vi "command_publisher.vi"() -> ()   [LabVIEW 2016]
uses:
  ts_sallv_exa/DataTypes/command_start.ctl
  ts_sallv_exa/SALLV_EXA.lvlib
panel:
  out "function return":i32
  out "waitComplete":cluster{"cmdSeqNum":i32, "timeout":u32}
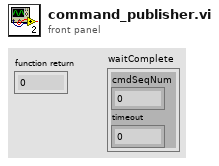
[diagram p1: front panel]
types:
  T1 = typedef "SALLV_EXA.lvlib/command_start.ctl" = cluster{"configuration":string}
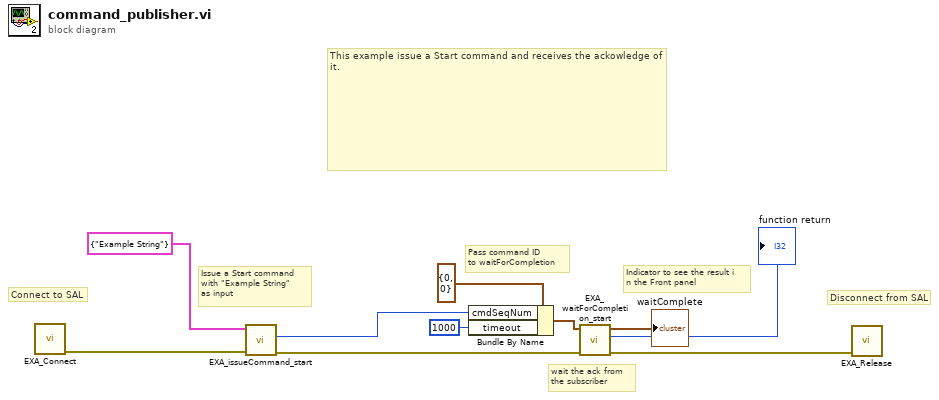
[diagram p0: block diagram]
diagram:
  # "wait the ack from \nthe subscriber"
  # "Indicator to see the result i\nn the Front panel"
  # "Pass command ID \nto waitForCompletion"
  # "Issue a Start command\nwith \"Example String\" \nas input"
  # "Disconnect from SAL"
  # "Connect to SAL"
  # "This example issue a Start command and receives the ackowledge of it."
  n1 = call "EXA_Connect.vi"() -> ("error out"=w3:errorcluster)  [unwired: 10 in, 1 out]
  n2 = call "EXA_issueCommand_start.vi"("error in (no error)"=w3, "command_start_Ctl"=T1 {"configuration"="Example String"}) -> ("error out"=w9:errorcluster, "function return"=w6:i32)  [unwired: 7 in, 1 out]
  n3 = Bundle By Name(cluster=cluster{"cmdSeqNum":i32, "timeout":u32} {"cmdSeqNum"=0, "timeout"=0} ("waitComplete_Ctl"), "cmdSeqNum"=w6, "timeout"=u32 1000) -> (w5:cluster{"cmdSeqNum":i32, "timeout":u32})
  n4 = call "EXA_waitForCompletion_start.vi"("error in (no error)"=w9, "waitComplete_Ctl"=w5) -> ("error out"=w8:errorcluster, "function return"=→"function return":i32, "waitComplete_Ctl out"=→"waitComplete":cluster{"cmdSeqNum":i32, "timeout":u32})  [unwired: 7 in]
  n5 = call "EXA_Release.vi"("error in (no error)"=w8) -> ()  [unwired: 9 in, 2 out]
